vi "PVCAM_StartCont.vi"(8 "error in (no error)":errorcluster, 10 "buffer":u8[](array[numeric]), 11 "hCam":i16) -> (0 "error out":errorcluster, 2 "return type":i16, 3 "ImageBuf":u8[](array[numeric]))   [LabVIEW 2021]
uses:
  pvcam64.dll
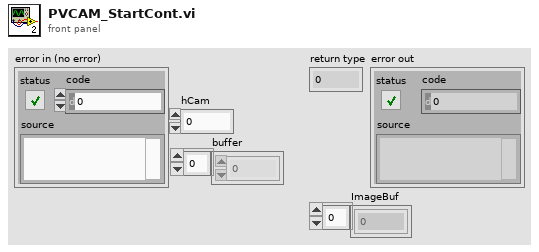
[diagram p1: front panel]
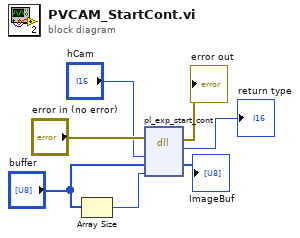
[diagram p0: block diagram]
diagram:
  n1 = Array Size(array="buffer") -> (size(s)=w1:i32)
  n2 = dll-call lib="pvcam64.dll" fn="pl_exp_start_cont"(error in="error in (no error)", "hCam"="hCam", "ImageBuf"="buffer", "size"=w1) -> (error out=→"error out":errorcluster, "return type"=→"return type":i16, "ImageBuf"=→"ImageBuf":u16[])  [unwired: 4 in, 1 out]
